vi "main_control.vi"(0 "VISA resource name":refnum<visa-resource-name>="COM6", 1 "baud rate":u32=9600, 2 "data bits":u16=8 min=5 max=8 step=1, 3 "parity":u16(ring) items=["None", "Odd", "Even", "Mark", "Space"], 4 "stop bits":u16(ring)=10 items=["1.0"=10, "1.5"=15, "2.0"=20], 6 "read":bool=TRUE, 7 "flow control":u16(ring) items=["None"=0, "XON/XOFF"=1, "RTS/CTS"=2, "DTR/DSR"=4]) -> (9 "read string":string, 10 "bytes read":u32)   [LabVIEW 2019]
doc: "The Basic Serial Read and Write example performs a Serial Port Read, a Serial Port Write, or a combination of these actions. The user selects the actions (read or write) on the front panel. If both are selected, the VI will write the data first, read data, and then close the VISA session that is opened to the port. This VI will wait until the specified number of bytes is received at the port. Only the number of bytes specified will be read.\n\nINSTRUCTIONS:\n1) Select the serial resource and configuration parameters (baud rate, data bits, parity, stop bits, flow control).\n2) Select the operations to be performed. \n3) Connect the serial port to your device. If no device is available, perform a loopback test by doing one of the following. Short pins 2 and 3 on a RS-232 cable or short pin 4 to pin 8 and pin 5 to pin 9 on a RS-485/422 cable. \n4) Run the VI to see the data read. (The \"read string\" will match the \"string to write\" if a loopback test was performed.)\n\nNote: The parameters set for the serial port must match the parameters of the connected instrument or device. In this example, the bytes to read parameter specifies the number of bytes that the serial port reads. If there were more bytes at the port than the number specified in bytes to read, those bytes would not be read. Also, if you specify to read more bytes than the number of bytes actually read, you might receive a timeout error message.\n\nOn the block diagram, the Configure Serial Port VI sets the configuration parameters. The front panel displays the controls used to configure the basic parameters, such as baud rate, data bits, and parity. Constants configure the other parameters the user probably does not need set. After the VISA Configure Serial Port VI opens the VISA session and configures the port, the VI passes the VISA resource name to other VIs that perform operations on that VISA resource. The VISA Write function sends a command to the serial device and the VISA Read function returns data based on the command. The VISA Close function then closes the reference to the serial device. It is important to close the reference; otherwise communication through with that port through protocols other than VISA might not be possible."
uses:
  <vilib>/Instr/_visa.llb/VISA Configure Serial Port (Instr).vi
  Keithley/Keithley 24XX/Public/Data/Read (Single Point).vi
  Keithley/Keithley 24XX/Keithley 24XX.lvlib
  DELTA ELEKTRONIKA SM Series/DELTA ELEKTRONIKA.lvlib
panel:
  in  "Current Limit (0A)":dbl format="%.2f"
  in  "Voltage Level (0.0 V)":dbl format="%.2f"
  in  "Stop Main":bool
  out "Actual Voltage Level (V)":dbl format="%.2f"
  out "Actual Current Limit (A)":dbl format="%.2f"
  out "Voltage Limit":bool
  out "Current Limit":bool
  in  "VISA resource name 5":refnum<visa-resource-name>
  out "Current Micro":sgl
  in  "Serial Configuration":T1={"Baud Rate"=9600, "Parity"=0, "Data Bits"=8, "Stop Bits"=10, "Flow Control"=1} {"Flow Control" items=["None", "XON/XOFF", "RTS/CTS", "XON/XOFF & RTS/CTS", "DTR/DSR", "XON/XOFF & DTR/DSR"]; "Stop Bits" items=["1.0"=10, "1.5"=15, "2.0"=20]; "Data Bits" items=["7"=7, "8"=8]; "Parity" items=["None", "Odd", "Even", "Mark", "Space"]; "Baud Rate" items=["300"=300, "600"=600, "1200"=1200, "2400"=2400, "4800"=4800, "9600"=9600, "19200"=19200]}
  in  "VISA resource name 4":refnum<visa-resource-name>="COM1"
  in  "Voltage Manual Range (1.0)":dbl=1.0
  in  "Current Manual Range (1.0)":dbl=1.0
  in  "Resistance Manual Range (1.0)":dbl=1.0
  in  "Enable Voltage Auto Range (T:Enable)":bool=TRUE
  in  "Enable Current Auto Range (T:Enable)":bool=TRUE
  in  "Enable Resistance Auto Range (T:Enable)":bool=TRUE
  in  "Output Level (0) 2":dbl
  in  "Compliance  Level (0.1) 2":dbl=0.1
  in  "Source Mode  (0: Voltage) 2":u16(ring) items=["Voltage", "Current"]
  out "Voltage 2":sgl
  out "Current 2":sgl
  out "Resistance":sgl
  in  "Set Value":bool
  out "relay TTi":errorcluster
  out "bytes read 3":u32
  out "read string 3":string
  in  "read 3":bool=TRUE
  in  "delay before read (ms) 3":u32=500
  in  "Combo Box 3":string(combo)
  in  "voltage or current 2":dbl
  out "string from combo 3":string
  in  "write 3":bool
  in  "flow control 3":u16(ring) items=["None"=0, "XON/XOFF"=1, "RTS/CTS"=2, "DTR/DSR"=4]
  in  "stop bits 3":u16(ring)=10 items=["1.0"=10, "1.5"=15, "2.0"=20]
  in  "parity 3":u16(ring) items=["None", "Odd", "Even", "Mark", "Space"]
  in  "data bits 3":u16=8 min=5 max=8 step=1
  in  "VISA resource name 3":refnum<visa-resource-name>="COM4"
  in  "baud rate 3":u32=9600
  out "LV TTi":errorcluster
  out "bytes read 2":u32
  out "read string 2":string
  in  "read 2":bool=TRUE
  in  "delay before read (ms) 2":u32=500
  in  "Combo Box 2":string(combo)
  in  "voltage or current":dbl
  out "string from combo 2":string
  in  "write 2":bool
  in  "flow control 2":u16(ring) items=["None"=0, "XON/XOFF"=1, "RTS/CTS"=2, "DTR/DSR"=4]
  in  "stop bits 2":u16(ring)=10 items=["1.0"=10, "1.5"=15, "2.0"=20]
  in  "parity 2":u16(ring) items=["None", "Odd", "Even", "Mark", "Space"]
  in  "data bits 2":u16=8 min=5 max=8 step=1
  in  "VISA resource name 2":refnum<visa-resource-name>="COM5"
  in  "baud rate 2":u32=9600
  in  "Table Control":string[][](table)
  in  "write":bool
  out "string from combo":string
  in  "Temperature":dbl
  in  "Combo Box":string(combo)
  out "Chiller":errorcluster
  out "N2 temperature > dew point + 2C":bool
  in  "File Path of rotonic datalog":path
  out "time humidity temporature dewpoint":string[](array[string])
  in  "Quit":bool
  in  "delay before read (ms)":u32=500
  # "Medical Chiller Interface\nCOM 6 is default"
  # "PSC488  powersupply Interface GPIB"
  # "TTi LV powersupply Interface\nCOM 5 is default"
  # "TTi LV powersupply Interface for the relay polarity control\nCOM 4 is default"
  # "Kethley powersupply Interface\nCOM 1 is default"
  # "µA"
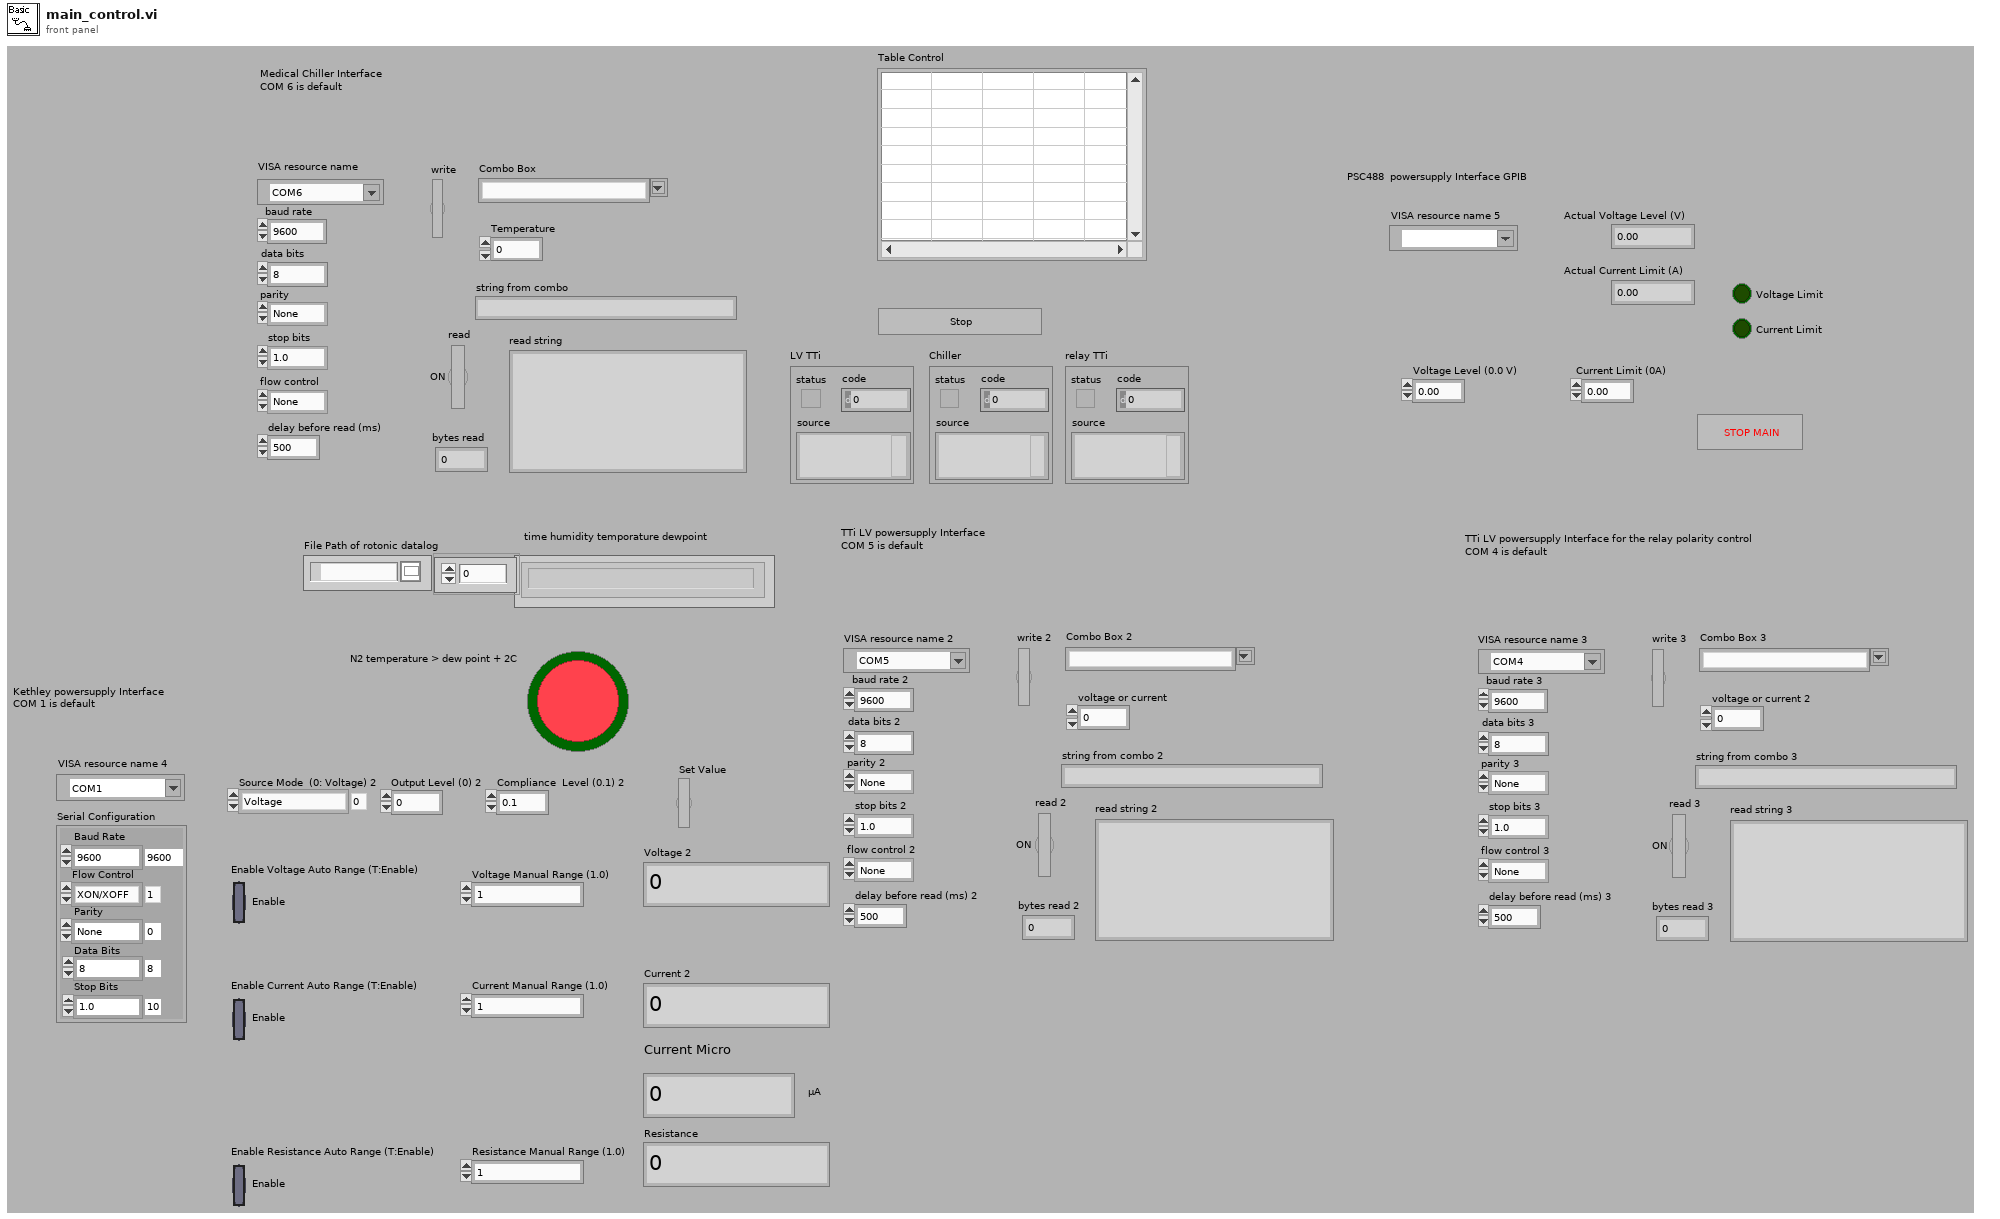
[diagram p1: front panel]
types:
  T1 = cluster{"Baud Rate":u32, "Parity":u16, "Data Bits":u16, "Stop Bits":u16, "Flow Control":u16}
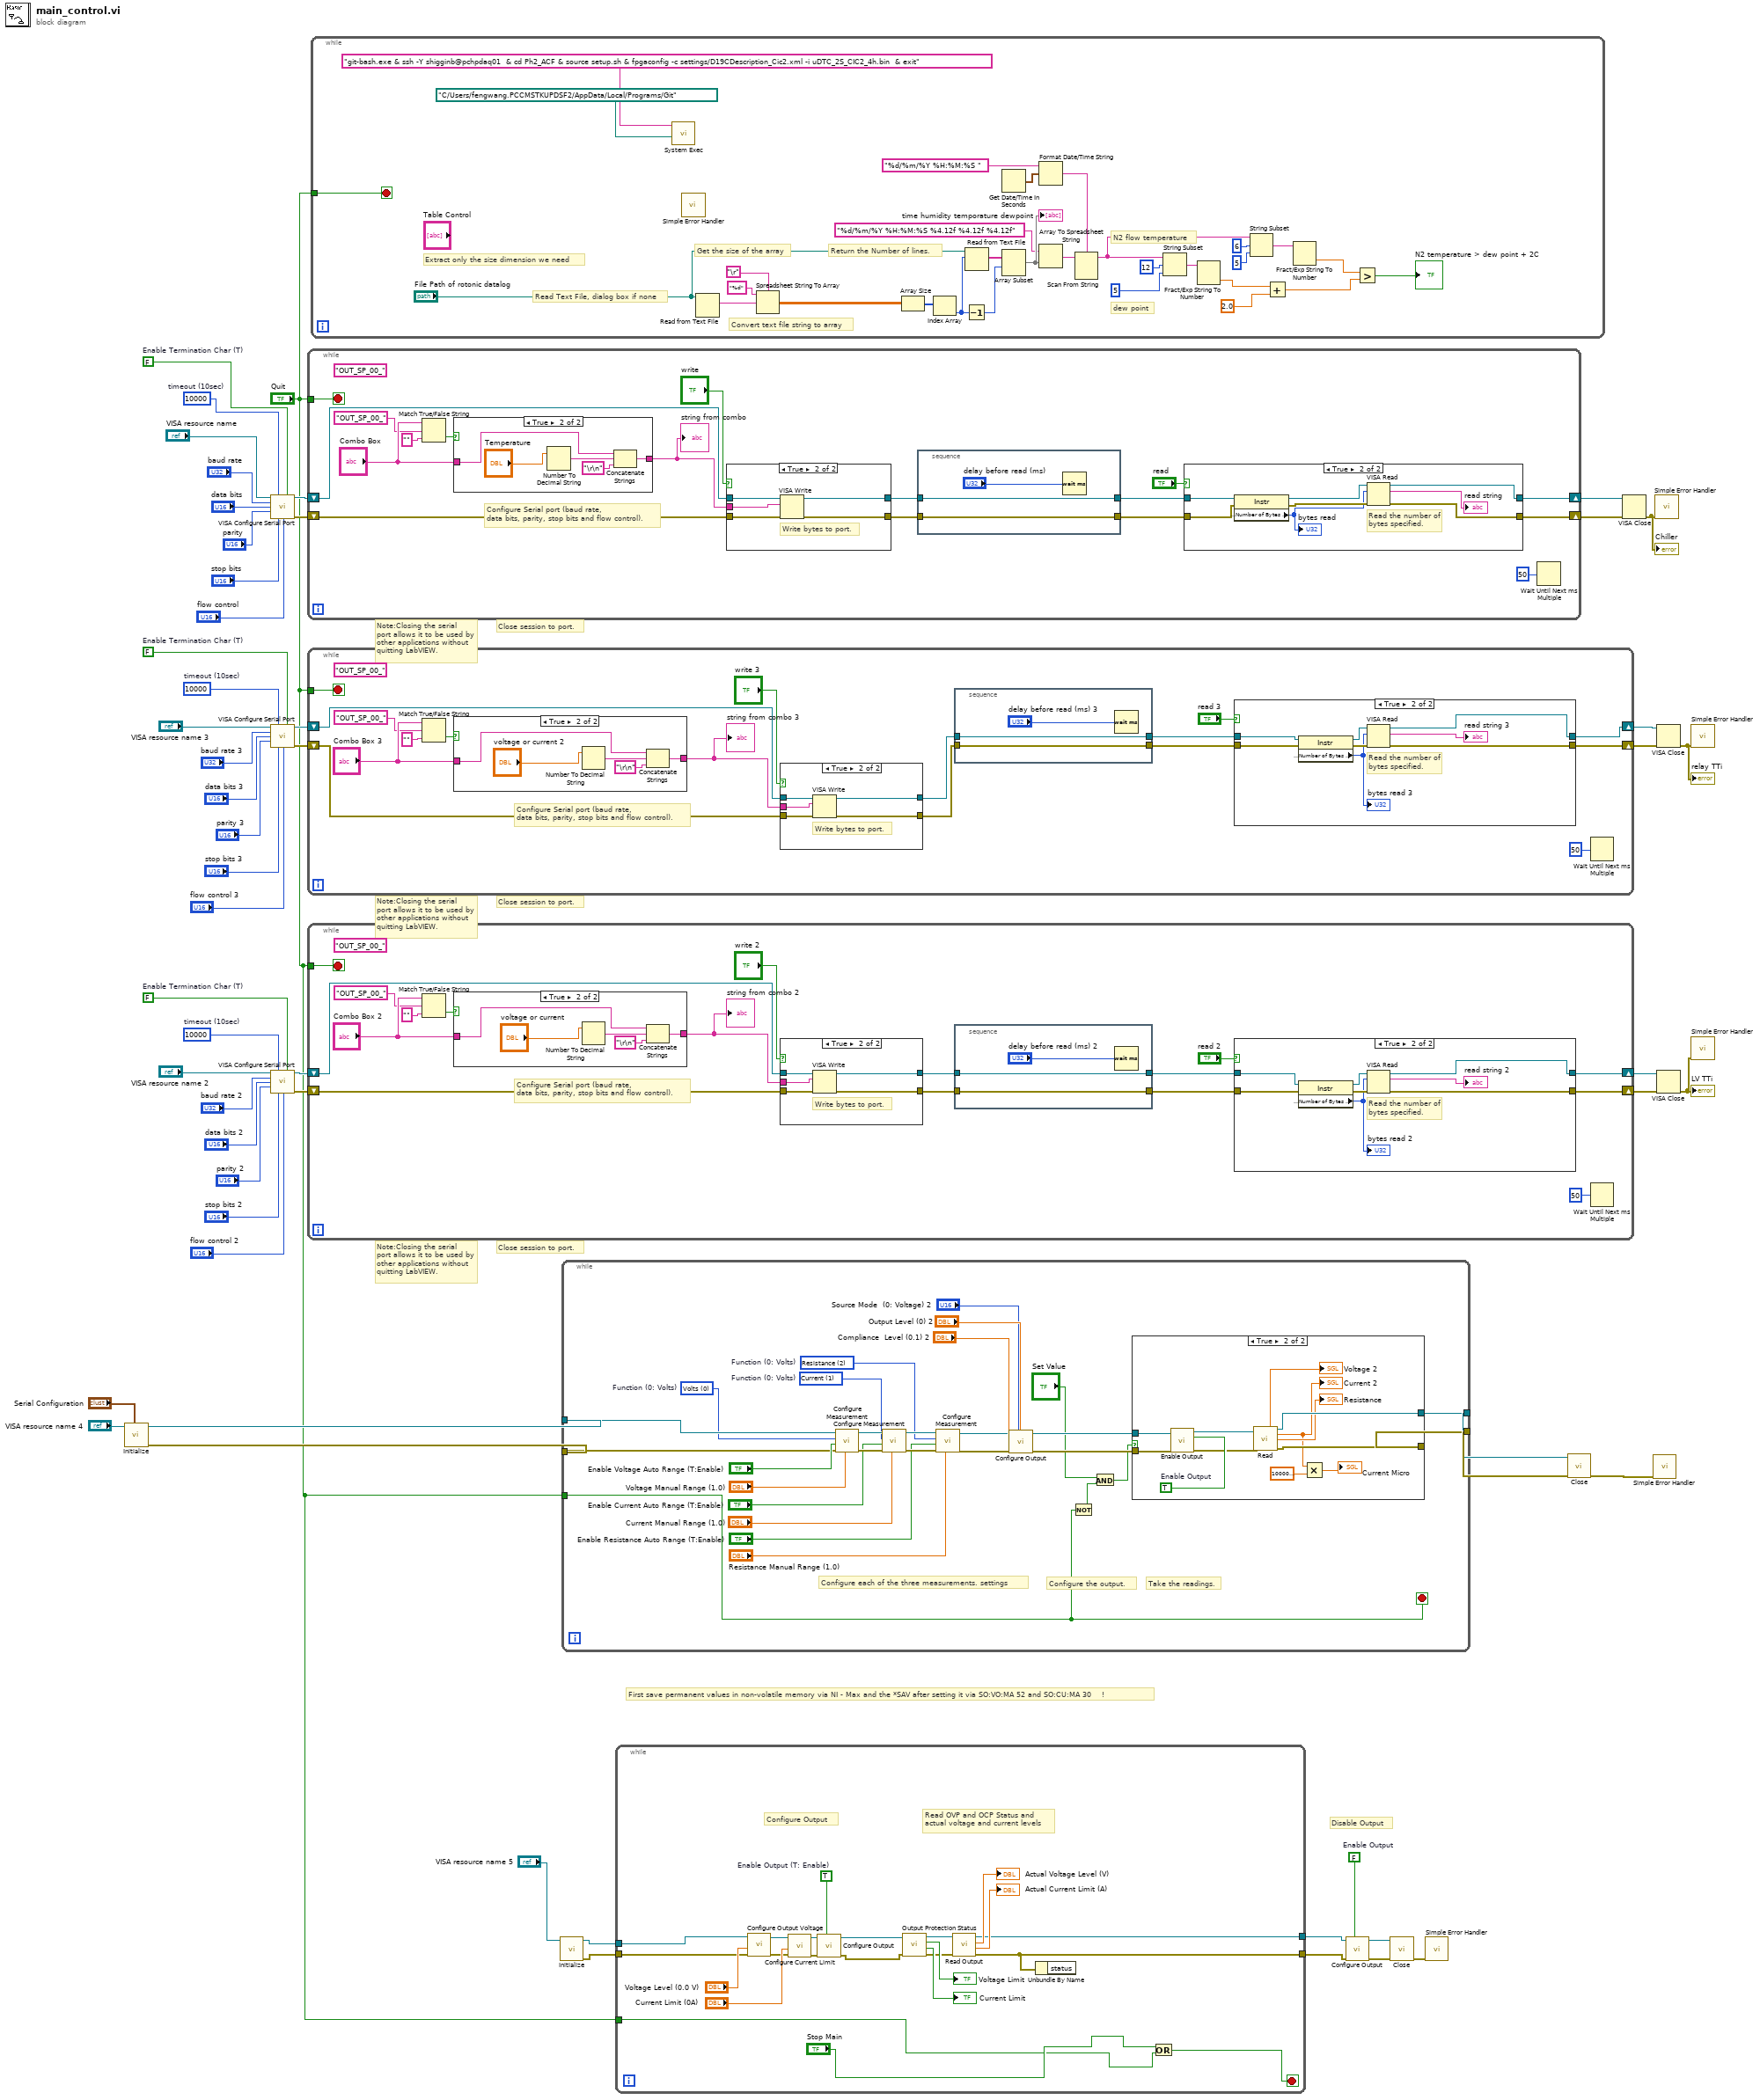
[diagram p0: block diagram]
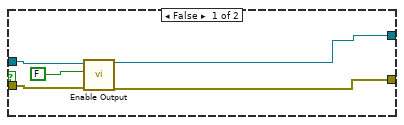
[diagram p2: hidden frame]
diagram:
  w4 = FALSE  # Enable Output
  w23 = FALSE  # Enable Termination Char (T)
  w24 = u32 10000  # timeout (10sec)
  w36 = FALSE  # Enable Termination Char (T)
  w37 = u32 10000  # timeout (10sec)
  w49 = FALSE  # Enable Termination Char (T)
  w50 = u32 10000  # timeout (10sec)
  # "Disable Output"
  # "First save permanent values in non-volatile memory via NI - Max and the *SAV after setting it via SO:VO:MA 52 and SO:CU:MA 30    !"
  # "Note:Closing the serial port allows it to be used by other applications without\nquitting LabVIEW."
  # "Close session to port."
  # "Note:Closing the serial port allows it to be used by other applications without\nquitting LabVIEW."
  # "Close session to port."
  # "Note:Closing the serial port allows it to be used by other applications without\nquitting LabVIEW."
  # "Close session to port."
  n1 = call "Initialize.vi"("Serial Configuration"="Serial Configuration", "VISA resource name"="VISA resource name 4") -> ("error out"=w15:errorcluster, "VISA resource name out"=w14:refnum<visa-resource-name>)  [unwired: 8 in]
  n2 = call-poly "VISA Configure Serial Port"("VISA resource name"="VISA resource name", "timeout (10sec)"=w50, "Enable Termination\nChar (T)"=w49, "baud rate (9600)"="baud rate", "data bits (8)"="data bits", "parity (0:none)"="parity", "stop bits (10: 1 bit)"="stop bits", "flow control (0:none)"="flow control") -> ("VISA resource name out"=w54:refnum<visa-resource-name>, "error out"=w45:errorcluster)  [unwired: 6 in]
  n3 = call-poly "VISA Configure Serial Port"("VISA resource name"="VISA resource name 3", "timeout (10sec)"=w24, "Enable Termination\nChar (T)"=w23, "baud rate (9600)"="baud rate 3", "data bits (8)"="data bits 3", "parity (0:none)"="parity 3", "stop bits (10: 1 bit)"="stop bits 3", "flow control (0:none)"="flow control 3") -> ("VISA resource name out"=w28:refnum<visa-resource-name>, "error out"=w19:errorcluster)  [unwired: 6 in]
  n4 = call-poly "VISA Configure Serial Port"("VISA resource name"="VISA resource name 2", "timeout (10sec)"=w37, "Enable Termination\nChar (T)"=w36, "baud rate (9600)"="baud rate 2", "data bits (8)"="data bits 2", "parity (0:none)"="parity 2", "stop bits (10: 1 bit)"="stop bits 2", "flow control (0:none)"="flow control 2") -> ("VISA resource name out"=w41:refnum<visa-resource-name>, "error out"=w32:errorcluster)  [unwired: 6 in]
  n5 = while {
    shift-right: [w70] -> w53
    shift-left: w45 -> [w72]
    shift-right: [w69] -> w52
    shift-left: w54 -> [w71]
    tunnel: "Quit" -> [w63]
    stop <- w63 stop-if-true
    (unwired) "OUT_SP_00_" ("format string")
    # "Configure Serial port (baud rate,\ndata bits, parity, stop bits and flow control)."
    n6 = Match True/False String(2:"" ("false string"), 3:"OUT_SP_00_" ("format string"), 4:"Combo Box") -> (0:w61:bool)  [unwired: 1 out]
    n7 = case shown="True" w61 {
      tunnel: [w74 w77] -> w58
      tunnel: "Combo Box" -> [w74 w76]
      frame False {
      }
      frame True {
        n8 = Number To Decimal String(number="Temperature") -> (decimal integer string=w79:string)  [unwired: 1 in]
        n9 = Concatenate Strings(w76, w79, "\r\n" ("string")) -> (w77:string)
      }
    }
    "string from combo" <- w58
    n10 = case shown="True" "write" {
      tunnel: [w84 w89] -> w68
      tunnel: w71 -> [w83 w88]
      tunnel: w72 -> [w84 w87]
      tunnel: [w83 w86] -> w66
      tunnel: w58 -> [_ w85]
      frame False {
      }
      frame True {
        # "Write bytes to port."
        n11 = VISA Write(VISA resource name=w88, write buffer=w85, error in (no error)=w87) -> (VISA resource name out=w86:refnum<visa-resource-name>, error out=w89:errorcluster)  [unwired: 1 out]
      }
    }
    n12 = stacked-sequence {
      tunnel: w68 -> [w82]
      tunnel: [w82] -> w67
      tunnel: w66 -> [w81]
      tunnel: [w81] -> w65
      frame #0 {
        n13 = Wait (ms)(milliseconds to wait="delay before read (ms)") -> ()  [unwired: 1 out]
      }
    }
    n14 = case shown="True" "read" {
      tunnel: w67 -> [w91 w95]
      tunnel: [w91 w99] -> w70
      tunnel: [w90 w98] -> w69
      tunnel: w65 -> [w90 w97]
      frame False {
      }
      frame True {
        # "Read the number of bytes specified."
        n15 = property class="Instr"(reference=w97, error in=w95) -> (reference out=w96:refnum<visa-resource-name>, error out=w94:errorcluster, "Serial Settings:Number of Bytes at Serial Port"=w93:u32)
        "bytes read" <- w93
        n16 = VISA Read(VISA resource name=w96, byte count=w93, error in (no error)=w94) -> (VISA resource name out=w98:refnum<visa-resource-name>, read buffer=→"read string":string, error out=w99:errorcluster)  [unwired: 1 out]
      }
    }
    n17 = Wait Until Next ms Multiple(millisecond multiple=u32 50) -> ()  [unwired: 1 out]
  }
  n18 = while {
    shift-right: [w113] -> w27
    shift-left: w19 -> [w115]
    shift-right: [w112] -> w26
    shift-left: w28 -> [w114]
    tunnel: "Quit" -> [w100]
    stop <- w100 stop-if-true
    (unwired) "OUT_SP_00_" ("format string")
    # "Configure Serial port (baud rate,\ndata bits, parity, stop bits and flow control)."
    n19 = Match True/False String(2:"" ("false string"), 3:"OUT_SP_00_" ("format string"), 4:"Combo Box 3") -> (0:w105:bool)  [unwired: 1 out]
    n20 = case shown="True" w105 {
      tunnel: [w117 w120] -> w102
      tunnel: "Combo Box 3" -> [w117 w119]
      frame False {
      }
      frame True {
        n21 = Number To Decimal String(number="voltage or current 2") -> (decimal integer string=w122:string)  [unwired: 1 in]
        n22 = Concatenate Strings(w119, w122, "\r\n" ("string")) -> (w120:string)
      }
    }
    "string from combo 3" <- w102
    n23 = case shown="True" "write 3" {
      tunnel: [w127 w132] -> w111
      tunnel: w114 -> [w126 w131]
      tunnel: w115 -> [w127 w130]
      tunnel: [w126 w129] -> w109
      tunnel: w102 -> [_ w128]
      frame False {
      }
      frame True {
        # "Write bytes to port."
        n24 = VISA Write(VISA resource name=w131, write buffer=w128, error in (no error)=w130) -> (VISA resource name out=w129:refnum<visa-resource-name>, error out=w132:errorcluster)  [unwired: 1 out]
      }
    }
    n25 = stacked-sequence {
      tunnel: w111 -> [w125]
      tunnel: [w125] -> w110
      tunnel: w109 -> [w124]
      tunnel: [w124] -> w108
      frame #0 {
        n26 = Wait (ms)(milliseconds to wait="delay before read (ms) 3") -> ()  [unwired: 1 out]
      }
    }
    n27 = case shown="True" "read 3" {
      tunnel: w110 -> [w134 w138]
      tunnel: [w134 w142] -> w113
      tunnel: [w133 w141] -> w112
      tunnel: w108 -> [w133 w140]
      frame False {
      }
      frame True {
        # "Read the number of bytes specified."
        n28 = property class="Instr"(reference=w140, error in=w138) -> (reference out=w139:refnum<visa-resource-name>, error out=w137:errorcluster, "Serial Settings:Number of Bytes at Serial Port"=w136:u32)
        "bytes read 3" <- w136
        n29 = VISA Read(VISA resource name=w139, byte count=w136, error in (no error)=w137) -> (VISA resource name out=w141:refnum<visa-resource-name>, read buffer=→"read string 3":string, error out=w142:errorcluster)  [unwired: 1 out]
      }
    }
    n30 = Wait Until Next ms Multiple(millisecond multiple=u32 50) -> ()  [unwired: 1 out]
  }
  n31 = while {
    shift-right: [w156] -> w40
    shift-left: w32 -> [w158]
    shift-right: [w155] -> w39
    shift-left: w41 -> [w157]
    tunnel: "Quit" -> [w143]
    stop <- w143 stop-if-true
    (unwired) "OUT_SP_00_" ("format string")
    # "Configure Serial port (baud rate,\ndata bits, parity, stop bits and flow control)."
    n32 = Match True/False String(2:"" ("false string"), 3:"OUT_SP_00_" ("format string"), 4:"Combo Box 2") -> (0:w148:bool)  [unwired: 1 out]
    n33 = case shown="True" w148 {
      tunnel: [w160 w163] -> w145
      tunnel: "Combo Box 2" -> [w160 w162]
      frame False {
      }
      frame True {
        n34 = Number To Decimal String(number="voltage or current") -> (decimal integer string=w165:string)  [unwired: 1 in]
        n35 = Concatenate Strings(w162, w165, "\r\n" ("string")) -> (w163:string)
      }
    }
    "string from combo 2" <- w145
    n36 = case shown="True" "write 2" {
      tunnel: [w170 w175] -> w154
      tunnel: w157 -> [w169 w174]
      tunnel: w158 -> [w170 w173]
      tunnel: [w169 w172] -> w152
      tunnel: w145 -> [_ w171]
      frame False {
      }
      frame True {
        # "Write bytes to port."
        n37 = VISA Write(VISA resource name=w174, write buffer=w171, error in (no error)=w173) -> (VISA resource name out=w172:refnum<visa-resource-name>, error out=w175:errorcluster)  [unwired: 1 out]
      }
    }
    n38 = stacked-sequence {
      tunnel: w154 -> [w168]
      tunnel: [w168] -> w153
      tunnel: w152 -> [w167]
      tunnel: [w167] -> w151
      frame #0 {
        n39 = Wait (ms)(milliseconds to wait="delay before read (ms) 2") -> ()  [unwired: 1 out]
      }
    }
    n40 = case shown="True" "read 2" {
      tunnel: w153 -> [w177 w181]
      tunnel: [w177 w185] -> w156
      tunnel: [w176 w184] -> w155
      tunnel: w151 -> [w176 w183]
      frame False {
      }
      frame True {
        # "Read the number of bytes specified."
        n41 = property class="Instr"(reference=w183, error in=w181) -> (reference out=w182:refnum<visa-resource-name>, error out=w180:errorcluster, "Serial Settings:Number of Bytes at Serial Port"=w179:u32)
        "bytes read 2" <- w179
        n42 = VISA Read(VISA resource name=w182, byte count=w179, error in (no error)=w180) -> (VISA resource name out=w184:refnum<visa-resource-name>, read buffer=→"read string 2":string, error out=w185:errorcluster)  [unwired: 1 out]
      }
    }
    n43 = Wait Until Next ms Multiple(millisecond multiple=u32 50) -> ()  [unwired: 1 out]
  }
  n44 = while {
    tunnel: "Quit" -> [w191]
    stop <- w191 stop-if-true
    # "dew point"
    # "N2 flow temperature"
    # "Convert text file string to array"
    # "Return the Number of lines."
    # "Extract only the size dimension we need"
    # "Get the size of the array"
    # "Read Text File, dialog box if none"
    n45 = call <vilib>:"System Exec.vi"("working directory"=path "C:/Users/fengwang.PCCMSTKUPDSF2/AppData/Local/Programs/Git", "command line"="git-bash.exe & ssh -Y shigginb@pchpdaq01  & cd Ph2_ACF & source setup.sh & fpgaconfig -c settings/D19CDescription_Cic2.xml -i uDTC_2S_CIC2_4h.bin  & exit") -> ()  [unwired: 6 in, 4 out]
    n46 = call <vilib>:"Simple Error Handler.vi"() -> ()  [unwired: 5 in, 5 out]
    n47 = Read from Text File(file (use dialog)="File Path of rotonic datalog") -> (text=w204:string)  [unwired: 1 in, 5 out]
    n48 = Spreadsheet String To Array(delimiter (Tab)="\r", format string="%d", spreadsheet string=w204) -> (array=w202:dbl[][])  [unwired: 1 out]
    n49 = Array Size(array=w202) -> (size(s)=w203:i32[])
    n50 = Index Array(array=w203) -> (element=w207:i32)  [unwired: 1 in]
    n51 = Decrement(x=w207) -> (x-1=w205:i32)
    n52 = Read from Text File(file (use dialog)="File Path of rotonic datalog", count=w207) -> (text=w208:string[])  [unwired: 1 in, 4 out]
    n53 = Get Date/Time In Seconds() -> (seconds since 1Jan1904=w200:timestamp)
    n54 = Array Subset(array=w208, index=w205) -> (w209:string[])  [unwired: 1 in]
    "time humidity temporature dewpoint" <- w209
    n55 = Format Date/Time String(time format string (%c)="%d/%m/%Y %H:%M:%S ", seconds (now)=w200) -> (date/time string=w201:string)  [unwired: 1 in]
    n56 = Array To Spreadsheet String(array=w209, 3:"%d/%m/%Y %H:%M:%S %4.12f %4.12f %4.12f" ("time format string (%c)")) -> (spreadsheet string=w210:string)  [unwired: 1 in]
    n57 = Scan From String(format string=w201, input string=w210) -> (remaining string=w211:string)  [unwired: 4 in, 2 out]
    n58 = String Subset(string=w211, offset (0)=12, length (rest)=5 ("length (rest)")) -> (substring=w213:string)
    n59 = Fract/Exp String To Number(string=w213) -> (number=w189:dbl)  [unwired: 3 in, 1 out]
    n60 = String Subset(string=w211, offset (0)=6, length (rest)=5 ("length (rest)")) -> (substring=w212:string)
    n61 = Add(x=w189, y=2.0) -> (x+y=w188:dbl)
    n62 = Fract/Exp String To Number(string=w212) -> (number=w214:dbl)  [unwired: 3 in, 1 out]
    n63 = Greater?(x=w214, y=w188) -> (0:→"N2 temperature > dew point + 2C":bool)
  }
  n64 = call "Initialize.vi"("VISA resource name"="VISA resource name 5") -> ("error out"=w9:errorcluster, "VISA resource name out"=w8:refnum<visa-resource-name>)  [unwired: 9 in]
  n65 = while {
    tunnel: w15 -> [w224]
    tunnel: w14 -> [w223]
    tunnel: [w220] -> w12
    tunnel: [w221] -> w11
    tunnel: "Quit" -> [w216]
    stop <- w216 stop-if-true
    w222 = u16 0 items=["Volts", "Current", "Resistance"]  # Function (0: Volts)
    w238 = u16 2 items=["Volts", "Current", "Resistance"]  # Function (0: Volts)
    w239 = u16 1 items=["Volts", "Current", "Resistance"]  # Function (0: Volts)
    # "Take the readings."
    # "Configure the output."
    # "Configure each of the three measurements. settings"
    n66 = call "Configure Measurement.vi"("Manual Range (1.0)"="Voltage Manual Range (1.0)", "error in (no error)"=w224, "Enable Auto Range (T:Enable)"="Enable Voltage Auto Range (T:Enable)", "Function (0: Volts)"=w222, "VISA resource name"=w223) -> ("error out"=w242:errorcluster, "VISA resource name out"=w243:refnum<visa-resource-name>)  [unwired: 5 in]
    n67 = call "Configure Measurement.vi"("Manual Range (1.0)"="Current Manual Range (1.0)", "error in (no error)"=w242, "Enable Auto Range (T:Enable)"="Enable Current Auto Range (T:Enable)", "Function (0: Volts)"=w239, "VISA resource name"=w243) -> ("error out"=w241:errorcluster, "VISA resource name out"=w240:refnum<visa-resource-name>)  [unwired: 5 in]
    n68 = call "Configure Measurement.vi"("Manual Range (1.0)"="Resistance Manual Range (1.0)", "error in (no error)"=w241, "Enable Auto Range (T:Enable)"="Enable Resistance Auto Range (T:Enable)", "Function (0: Volts)"=w238, "VISA resource name"=w240) -> ("error out"=w227:errorcluster, "VISA resource name out"=w226:refnum<visa-resource-name>)  [unwired: 5 in]
    n69 = call "Configure Output.vi"("Source Mode  (0: Voltage)"="Source Mode  (0: Voltage) 2", "error in (no error)"=w227, "Compliance  Level (0.1)"="Compliance  Level (0.1) 2", "Output Level (0)"="Output Level (0) 2", "VISA resource name"=w226) -> ("error out"=w228:errorcluster, "VISA resource name out"=w229:refnum<visa-resource-name>)  [unwired: 5 in]
    n70 = Not(x=w216) -> (.not. x?=w219:bool)
    n71 = And(x="Set Value", y=w219) -> (x .and. y?=w217:bool)
    n72 = case shown="True" w217 {
      tunnel: w229 -> [w248 w260]
      tunnel: w228 -> [w247 w259]
      tunnel: [w245 w255] -> w221
      tunnel: [w244 w254] -> w220
      frame False {
        n73 = call "Enable Output.vi"("error in (no error)"=w247, "Enable Output (T: Enable)"=FALSE, "VISA resource name"=w248) -> ("error out"=w244:errorcluster, "VISA resource name out"=w245:refnum<visa-resource-name>)  [unwired: 7 in]
      }
      frame True {
        w258 = TRUE  # Enable Output
        n74 = call "Enable Output.vi"("error in (no error)"=w259, "Enable Output (T: Enable)"=w258, "VISA resource name"=w260) -> ("error out"=w256:errorcluster, "VISA resource name out"=w257:refnum<visa-resource-name>)  [unwired: 7 in]
        n75 = call-poly "Read.vi"("VISA resource name"=w257, "error in (no error)"=w256) -> ("Voltage"=→"Voltage 2":sgl, "VISA resource name out"=w255:refnum<visa-resource-name>, "Current"=w251:sgl, "Resistance"=→"Resistance":sgl, "error out"=w254:errorcluster)  [unwired: 7 in, 2 out]
        "Current 2" <- w251
        n76 = Multiply(x=w251, y=sgl 1000000.0) -> (x*y=→"Current Micro":sgl)
      }
    }
  }
  n77 = while {
    tunnel: w9 -> [w275]
    tunnel: w8 -> [w274]
    tunnel: [w265] -> w3
    tunnel: [w264] -> w2
    tunnel: "Quit" -> [w261]
    stop <- w262 stop-if-true
    w279 = TRUE  # Enable Output (T: Enable)
    # "Read OVP and OCP Status and\nactual voltage and current levels"
    # "Configure Output"
    n78 = call "Configure Output Voltage.vi"("error in (no error)"=w275, "Set Voltage(0.0 V)"="Voltage Level (0.0 V)", "VISA resource name"=w274) -> ("error out"=w278:errorcluster, "VISA resource name out"=w277:refnum<visa-resource-name>)  [unwired: 7 in]
    n79 = call "Configure Current Limit.vi"("error in (no error)"=w278, "Current Limit (0.0 A)"="Current Limit (0A)", "VISA resource name"=w277) -> ("error out"=w281:errorcluster, "VISA resource name out"=w282:refnum<visa-resource-name>)  [unwired: 7 in]
    n80 = call "Configure Output.vi"("Enable Output (T: Enable)"=w279, "error in (no error)"=w281, "VISA resource name"=w282) -> ("error out"=w267:errorcluster, "VISA resource name out"=w266:refnum<visa-resource-name>)  [unwired: 7 in]
    n81 = call "Output Protection Status.vi"("error in (no error)"=w267, "VISA resource name"=w266) -> ("error out"=w269:errorcluster, "OCP Tripped?"=→"Current Limit":bool, "OVP Tripped?"=→"Voltage Limit":bool, "VISA resource name out"=w268:refnum<visa-resource-name>)  [unwired: 6 in]
    n82 = call "Read Output.vi"("error in (no error)"=w269, "VISA resource name"=w268) -> ("error out"=w264:errorcluster, "Actual Current Level (A)"=→"Actual Current Limit (A)":dbl, "Actual Voltage Level (V)"=→"Actual Voltage Level (V)":dbl, "VISA resource name out"=w265:refnum<visa-resource-name>)  [unwired: 6 in]
    n83 = Unbundle By Name(w264) -> ()  [unwired: 1 out]
    n84 = Or(x="Stop Main", y=w261) -> (x .or. y?=w262:bool)
  }
  n85 = call "Configure Output.vi"("Enable Output (T: Enable)"=w4, "error in (no error)"=w2, "VISA resource name"=w3) -> ("error out"=w6:errorcluster, "VISA resource name out"=w5:refnum<visa-resource-name>)  [unwired: 7 in]
  n86 = call "Close.vi"("error in (no error)"=w6, "VISA resource name"=w5) -> ("error out"=w7:errorcluster)  [unwired: 9 in]
  n87 = call <vilib>:"Simple Error Handler.vi"("error in (no error)"=w7) -> ()  [unwired: 4 in, 5 out]
  n88 = call "Close.vi"("error in (no error)"=w12, "VISA resource name"=w11) -> ("error out"=w13:errorcluster)  [unwired: 9 in]
  n89 = VISA Close(VISA resource name=w52, error in (no error)=w53) -> (error out=w44:errorcluster)
  "Chiller" <- w44
  n90 = call <vilib>:"Simple Error Handler.vi"("error in (no error)"=w13) -> ()  [unwired: 4 in, 5 out]
  n91 = call <vilib>:"Simple Error Handler.vi"("error in (no error)"=w44) -> ()  [unwired: 4 in, 5 out]
  n92 = VISA Close(VISA resource name=w26, error in (no error)=w27) -> (error out=w18:errorcluster)
  "relay TTi" <- w18
  n93 = VISA Close(VISA resource name=w39, error in (no error)=w40) -> (error out=w31:errorcluster)
  "LV TTi" <- w31
  n94 = call <vilib>:"Simple Error Handler.vi"("error in (no error)"=w18) -> ()  [unwired: 4 in, 5 out]
  n95 = call <vilib>:"Simple Error Handler.vi"("error in (no error)"=w31) -> ()  [unwired: 4 in, 5 out]
